vi "EtherNet CIP Write_core.vi"(0 "Connection Cluster":T3={"TCP Connection"=refnum, "Session"=[], "EtherNet/IP Device Address"="172.20.37.243"} {"Session" format="0x%02x"}, 1 "Tag":string, 2 "SINT Array":u8[](array[numeric]), 3 "INT Array":u16[](array[numeric]), 4 "DINT Array":u32[](array[numeric]), 5 "error in":errorcluster, 6 "BOOL Array":bool[](array[boolean]), 7 "REAL Array":sgl[](array[numeric]), 8 "BOOL":bool, 9 "CONTROL/TIMER/COUNTER":T1, 10 "Datatype":T2(ring)) -> (14 "Connection Cluster Out":T3, 19 "error out":errorcluster)   [LabVIEW 2012]
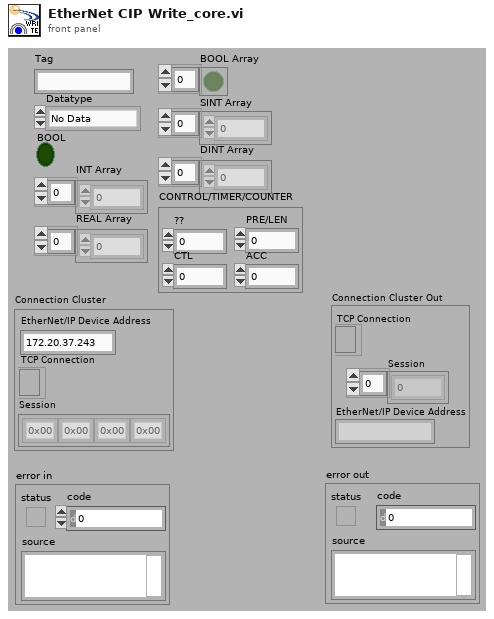
[diagram p1: front panel]
types:
  T1 = cluster{"??":u16, "CTL":u32, "PRE/LEN":u32, "ACC":u32}
  T2 = enum16{"No Data", "BOOL", "BIT Array", "SINT", "INT", "DINT", "REAL", "TIMER/CONTROL/COUNTER"}
  T3 = cluster{"TCP Connection":refnum<k5>, "Session":u8[], "EtherNet/IP Device Address":string}
  T4 = enum16{"Standard", "Buffered", "CRLF", "Immediate"}
  T5 = enum16{"Success", "Unknown Error", "Bad Symbolic Representation", "Item Not Found", "Partial Read", "Error Processing Attribute", "Incorrect/Insufficient Param", "Insufficient Attribute", "Bad Symbolic Length", "Out Of Bound", "Type Mismatch", "Offset Out Of Bound"}
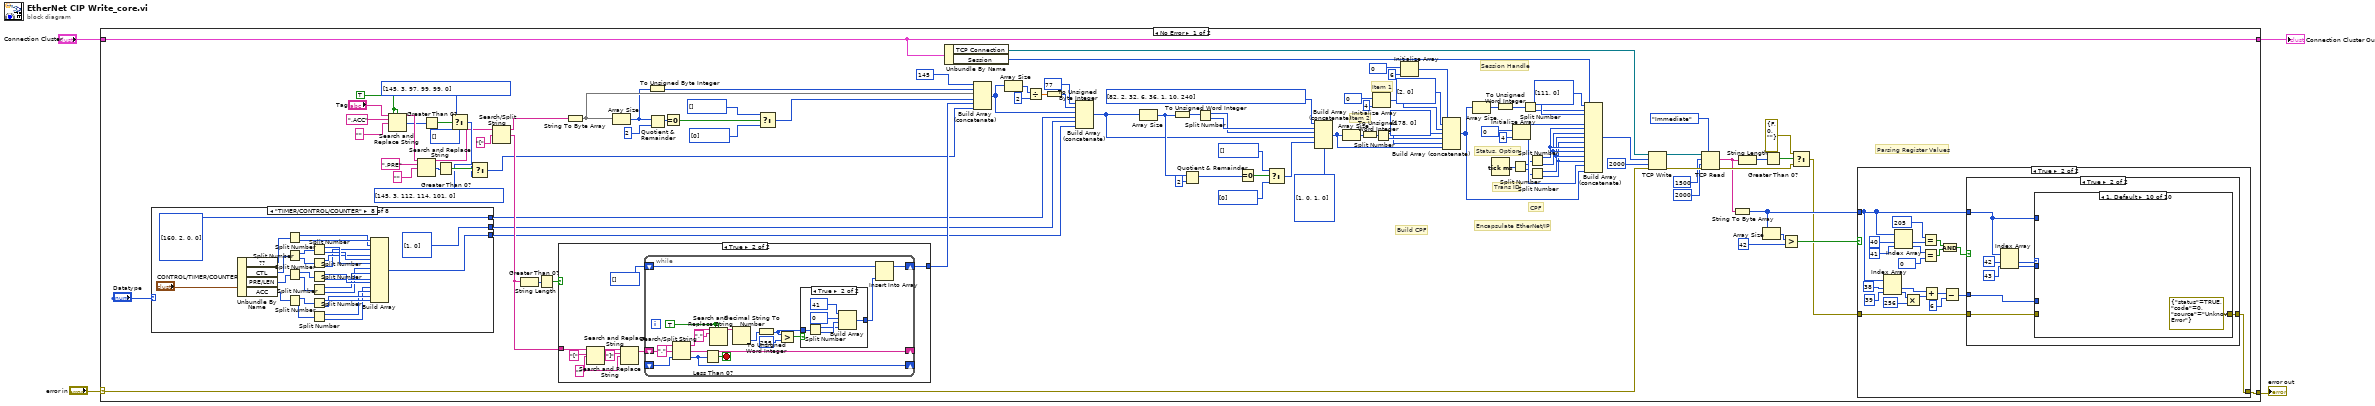
[diagram p0: block diagram]
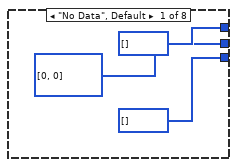
[diagram p2: hidden frame]
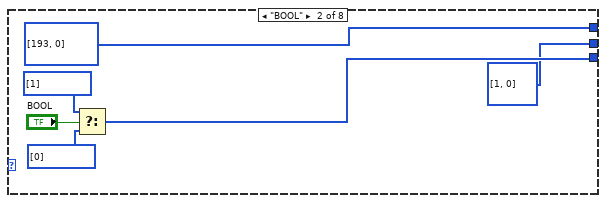
[diagram p3: hidden frame]
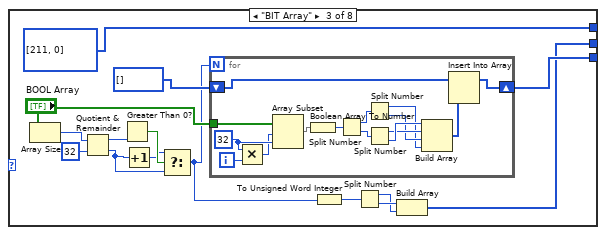
[diagram p4: hidden frame]
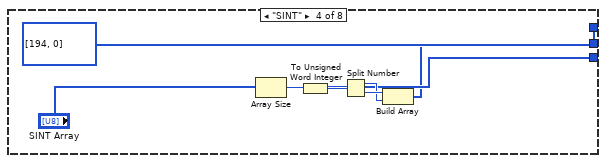
[diagram p5: hidden frame]
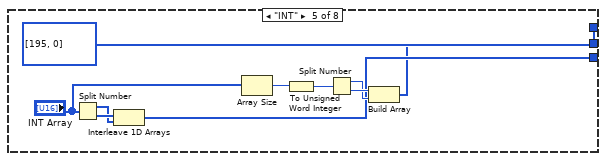
[diagram p6: hidden frame]
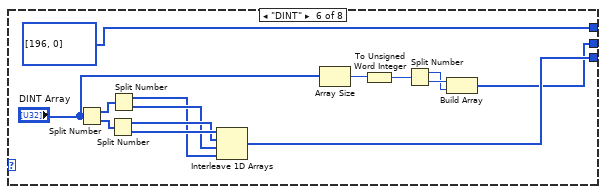
[diagram p7: hidden frame]
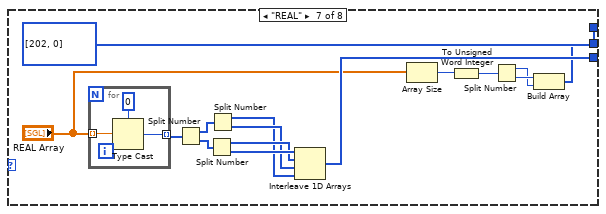
[diagram p8: hidden frame]
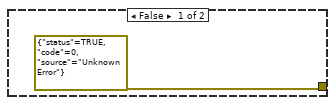
[diagram p9: hidden frame]
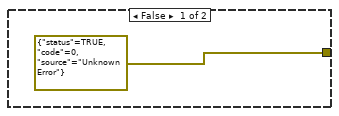
[diagram p10: hidden frame]
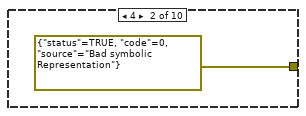
[diagram p12: hidden frame]
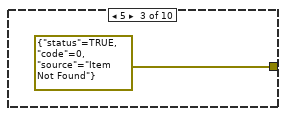
[diagram p13: hidden frame]
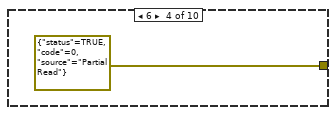
[diagram p14: hidden frame]
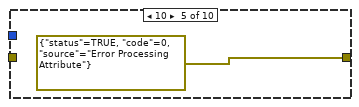
[diagram p15: hidden frame]
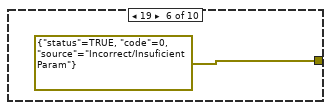
[diagram p16: hidden frame]
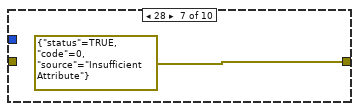
[diagram p17: hidden frame]
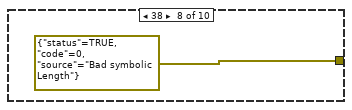
[diagram p18: hidden frame]
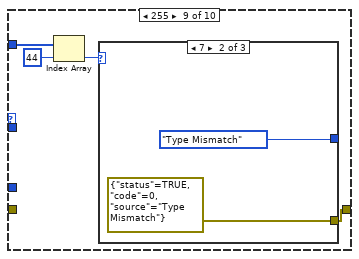
[diagram p19: hidden frame]
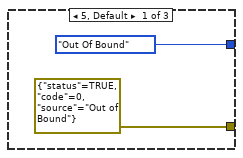
[diagram p20: hidden frame]
diagram:
  n1 = case shown="No Error" "error in" {
    selector: "error in" -> [w6 w315]
    tunnel: "Connection Cluster" -> [w5 w314]
    tunnel: [w8 w315] -> w4
    tunnel: [w5 w314] -> w1
    frame No Error {
      w61 = TRUE ("replace all? (F)")
      # "Parsing Register Values"
      # "Build CPF"
      # "Trans ID"
      # "CPF"
      # "Status, Option"
      # "Session Handle"
      # "Item 2"
      # "Item 1"
      # "Encapsulate EtherNet/IP"
      n2 = case shown="\"TIMER/CONTROL/COUNTER\"" "Datatype" {
        tunnel: [u8[] [] ("SINT Array") w119 w127 "SINT Array" w160 w174 w184 w200] -> w13
        tunnel: [u8[] [] u8[] [193, 0] u8[] [211, 0] u8[] [194, 0] u8[] [195, 0] u8[] [196, 0] u8[] [202, 0] u8[] [160, 2, 0, 0]] -> w14
        tunnel: [u8[] [0, 0] u8[] [1, 0] w123 w151 w159 w173 w183 u8[] [1, 0]] -> w12
        frame "No Data", Default {
        }
        frame "BOOL" {
          n3 = Select(t=u8[] [1], s="BOOL", f=u8[] [0]) -> (s? t:f=w119:u8[])
        }
        frame "BIT Array" {
          n4 = Array Size(array="BOOL Array") -> (size(s)=w122:i32)
          n5 = Quotient & Remainder(x=w122, y=32) -> (x-y*floor(x/y)=w133:i32, floor(x/y)=w131:i32)
          n6 = Greater Than 0?(x=w133) -> (x > 0?=w132:bool)
          n7 = Increment(x=w131) -> (x+1=w130:i32)
          n8 = Select(t=w130, s=w132, f=w131) -> (s? t:f=w121:i32)
          n9 = for {
            N: w121 -> [_]
            tunnel: "BOOL Array" -> [w150]
            shift-right: [w136] -> w127
            shift-left: u8[] [] -> [w138]
            i -> [w149]
            w148 = 32 ("length")
            n10 = Multiply(x=w148, y=w149) -> (x*y=w147:i32)
            n11 = Array Subset(array=w150, index=w147, length=w148) -> (w146:bool[])
            n12 = Boolean Array To Number(Boolean array=w146) -> (number=w145:u32)
            n13 = Split Number(x=w145) -> (hi(x)=w144:u16, lo(x)=w143:u16)
            n14 = Split Number(x=w144) -> (hi(x)=w139:u8, lo(x)=w140:u8)
            n15 = Split Number(x=w143) -> (hi(x)=w141:u8, lo(x)=w142:u8)
            n16 = Build Array(w142, w141, w140, w139) -> (w137:u8[])
            n17 = Insert Into Array(array=w138, new element=w137) -> (w136:u8[])  [unwired: 1 in]
          }
          n18 = To Unsigned Word Integer(number=w121) -> (unsigned 16bit integer=w126:u16)
          n19 = Split Number(x=w126) -> (hi(x)=w124:u8, lo(x)=w125:u8)
          n20 = Build Array(w125, w124) -> (w123:u8[])
        }
        frame "SINT" {
          n21 = Array Size(array="SINT Array") -> (size(s)=w156:i32)
          n22 = To Unsigned Word Integer(number=w156) -> (unsigned 16bit integer=w155:u16)
          n23 = Split Number(x=w155) -> (hi(x)=w153:u8, lo(x)=w154:u8)
          n24 = Build Array(w154, w153) -> (w151:u8[])
        }
        frame "INT" {
          n25 = Split Number(x="INT Array") -> (hi(x)=w165:u8[], lo(x)=w166:u8[])
          n26 = Interleave 1D Arrays(w166, w165) -> (w160:u8[])
          n27 = Array Size(array="INT Array") -> (size(s)=w164:i32)
          n28 = To Unsigned Word Integer(number=w164) -> (unsigned 16bit integer=w163:u16)
          n29 = Split Number(x=w163) -> (hi(x)=w161:u8, lo(x)=w162:u8)
          n30 = Build Array(w162, w161) -> (w159:u8[])
        }
        frame "DINT" {
          n31 = Split Number(x="DINT Array") -> (hi(x)=w180:u16[], lo(x)=w181:u16[])
          n32 = Split Number(x=w181) -> (hi(x)=w170:u8[], lo(x)=w171:u8[])
          n33 = Split Number(x=w180) -> (hi(x)=w168:u8[], lo(x)=w169:u8[])
          n34 = Interleave 1D Arrays(w171, w170, w169, w168) -> (w174:u8[])
          n35 = Array Size(array="DINT Array") -> (size(s)=w178:i32)
          n36 = To Unsigned Word Integer(number=w178) -> (unsigned 16bit integer=w177:u16)
          n37 = Split Number(x=w177) -> (hi(x)=w175:u8, lo(x)=w176:u8)
          n38 = Build Array(w176, w175) -> (w173:u8[])
        }
        frame "REAL" {
          n39 = for {
            tunnel: "REAL Array" -> [w198] mode=indexing
            tunnel: [w197] -> w190 mode=indexing
            n40 = Type Cast(type=u32 0, x=w198) -> (*(type *) &x=w197:u32)
          }
          n41 = Split Number(x=w190) -> (hi(x)=w195:u16[], lo(x)=w196:u16[])
          n42 = Split Number(x=w196) -> (hi(x)=w193:u8[], lo(x)=w194:u8[])
          n43 = Split Number(x=w195) -> (hi(x)=w191:u8[], lo(x)=w192:u8[])
          n44 = Interleave 1D Arrays(w194, w193, w192, w191) -> (w184:u8[])
          n45 = Array Size(array="REAL Array") -> (size(s)=w188:i32)
          n46 = To Unsigned Word Integer(number=w188) -> (unsigned 16bit integer=w187:u16)
          n47 = Split Number(x=w187) -> (hi(x)=w185:u8, lo(x)=w186:u8)
          n48 = Build Array(w186, w185) -> (w183:u8[])
        }
        frame "TIMER/CONTROL/COUNTER" {
          n49 = Unbundle By Name("CONTROL/TIMER/COUNTER") -> ("??"=w225:u16, "CTL"=w224:u32, "PRE/LEN"=w223:u32, "ACC"=w222:u32)
          n50 = Split Number(x=w225) -> (hi(x)=w214:u8, lo(x)=w215:u8)
          n51 = Split Number(x=w224) -> (hi(x)=w221:u16, lo(x)=w220:u16)
          n52 = Split Number(x=w223) -> (hi(x)=w219:u16, lo(x)=w218:u16)
          n53 = Split Number(x=w222) -> (hi(x)=w217:u16, lo(x)=w216:u16)
          n54 = Split Number(x=w221) -> (hi(x)=w213:u8, lo(x)=w212:u8)
          n55 = Split Number(x=w220) -> (hi(x)=w211:u8, lo(x)=w210:u8)
          n56 = Split Number(x=w219) -> (hi(x)=w209:u8, lo(x)=w208:u8)
          n57 = Split Number(x=w218) -> (hi(x)=w207:u8, lo(x)=w206:u8)
          n58 = Split Number(x=w217) -> (hi(x)=w205:u8, lo(x)=w204:u8)
          n59 = Split Number(x=w216) -> (hi(x)=w203:u8, lo(x)=w202:u8)
          n60 = Build Array(w215, w214, w210, w211, w212, w213, w206, w207, w208, w209, w202, w203, w204, w205) -> (w200:u8[])
        }
      }
      n61 = Search and Replace String(replace all?=w61, case sensitive?=w61, input string="Tag", search string=".ACC", replace string="" ("replace string (\"\")")) -> (result string=w58:string, number of replacements=w57:i32)  [unwired: 3 in, 2 out]
      n62 = Search and Replace String(input string=w58, search string=".PRE", replace string="" ("replace string (\"\")")) -> (result string=w48:string, number of replacements=w56:i32)  [unwired: 5 in, 2 out]
      n63 = Greater Than 0?(x=w57) -> (x > 0?=w55:bool)
      n64 = Greater Than 0?(x=w56) -> (x > 0?=w54:bool)
      n65 = Select(t=u8[] [145, 3, 97, 99, 99, 0], s=w55, f=u8[] []) -> (s? t:f=w51:u8[])
      n66 = Select(t=u8[] [145, 3, 112, 114, 101, 0], s=w54, f=w51) -> (s? t:f=w26:u8[])
      n67 = Search/Split String(string=w48, search string/char (-)="[") -> (substring before match=w47:string, match + rest of string=w28:string)  [unwired: 1 in, 1 out]
      n68 = String Length(string=w28) -> (length=w30:i32)
      n69 = Greater Than 0?(x=w30) -> (x > 0?=w29:bool)
      n70 = case shown="True" w29 {
        tunnel: w28 -> [_ w280]
        tunnel: [u8[] [] w279] -> w27
        frame False {
        }
        frame True {
          w283 = "" ("replace string (\"\")")
          n71 = Search and Replace String(input string=w280, search string="[", replace string=w283) -> (result string=w285:string)  [unwired: 5 in, 3 out]
          n72 = Search and Replace String(input string=w285, search string="]", replace string=w283) -> (result string=w282:string)  [unwired: 5 in, 3 out]
          n73 = while {
            shift-right: [w296] -> _
            shift-left: _ -> [w303]
            shift-right: [w301] -> _
            shift-left: w282 -> [w302]
            shift-right: [w288] -> w279
            shift-left: u8[] [] -> [w290]
            stop <- w297 stop-if-true
            w295 = TRUE ("replace all? (F)")
            n74 = Search/Split String(string=w302, search string/char (-)=",", offset (0)=w303) -> (substring before match=w299:string, match + rest of string=w301:string, offset of match=w296:i32)
            n75 = Less Than 0?(x=w296) -> (x < 0?=w297:bool)
            n76 = Search and Replace String(replace all?=w295, case sensitive?=w295, input string=w299, search string=",") -> (result string=w294:string)  [unwired: 4 in, 3 out]
            n77 = Decimal String To Number(string=w294) -> (number=w291:i32)  [unwired: 2 in, 1 out]
            n78 = To Unsigned Word Integer(number=w291) -> (unsigned 16bit integer=w287:u16)
            n79 = Greater?(x=w287, y=u16 255) -> (0:w292:bool)
            n80 = case shown="True" w292 {
              tunnel: w287 -> [w307 w313]
              tunnel: [w304 w308] -> w289
              frame False {
                n81 = To Unsigned Byte Integer(number=w307) -> (unsigned 8bit integer=w306:u8)
                n82 = Build Array(u8 40 ("Status"), w306) -> (w304:u8[])
              }
              frame True {
                n83 = Split Number(x=w313) -> (hi(x)=w311:u8, lo(x)=w312:u8)
                n84 = Build Array(u8 41 ("Status"), u8 0 ("Status"), w312, w311) -> (w308:u8[])
              }
            }
            n85 = Insert Into Array(array=w290, new element=w289) -> (w288:u8[])  [unwired: 1 in]
          }
        }
      }
      n86 = String To Byte Array(string=w47) -> (unsigned byte array=w45:u8[])
      n87 = Array Size(array=w45) -> (size(s)=w32:i32)
      n88 = To Unsigned Byte Integer(number=w32) -> (unsigned 8bit integer=w44:u8)
      n89 = Quotient & Remainder(x=w32, y=2) -> (x-y*floor(x/y)=w34:i32)  [unwired: 1 out]
      n90 = Equal To 0?(x=w34) -> (x = 0?=w37:bool)
      n91 = Select(t=u8[] [], s=w37, f=u8[] [0]) -> (s? t:f=w31:u8[])
      n92 = Unbundle By Name(w5) -> ("TCP Connection"=w108:refnum<k5>, "Session"=w94:u8[])
      n93 = Build Array (concatenate)(u8 145 ("Status"), w44, w45, w31, w27, w26) -> (w23:u8[])
      n94 = Array Size(array=w23) -> (size(s)=w11:i32)
      n95 = Divide(x=w11, y=u8 2) -> (x/y=w9:dbl)
      n96 = To Unsigned Byte Integer(number=w9) -> (unsigned 8bit integer=w24:u8)
      n97 = Build Array (concatenate)(u8 77 ("Status"), w24, w23, w14, w12, w13) -> (w22:u8[])
      n98 = Array Size(array=w22) -> (size(s)=w38:i32)
      n99 = To Unsigned Word Integer(number=w38) -> (unsigned 16bit integer=w106:u16)
      n100 = Quotient & Remainder(x=w38, y=2) -> (x-y*floor(x/y)=w65:i32)  [unwired: 1 out]
      n101 = Split Number(x=w106) -> (hi(x)=w104:u8, lo(x)=w105:u8)
      n102 = Equal To 0?(x=w65) -> (x = 0?=w40:bool)
      n103 = Select(t=u8[] [], s=w40, f=u8[] [0]) -> (s? t:f=w39:u8[])
      n104 = Build Array (concatenate)(u8[] [82, 2, 32, 6, 36, 1, 10, 240], w105, w104, w22, w39, u8[] [1, 0, 1, 0]) -> (w67:u8[])
      n105 = Array Size(array=w67) -> (size(s)=w71:i32)
      n106 = To Unsigned Word Integer(number=w71) -> (unsigned 16bit integer=w72:u16)
      n107 = Initialize Array(u8 0 ("Status"), 4 ("dimension size")) -> (w69:u8[])
      n108 = Split Number(x=w72) -> (hi(x)=w68:u8, lo(x)=w70:u8)
      n109 = Initialize Array(u8 0 ("Status"), 6 ("dimension size")) -> (w75:u8[])
      n110 = Build Array (concatenate)(w75, u8[] [2, 0], w69, u8[] [178, 0], w70, w68, w67) -> (w21:u8[])
      n111 = Array Size(array=w21) -> (size(s)=w100:i32)
      n112 = Tick Count (ms)() -> (millisecond timer value=w93:u32)
      n113 = To Unsigned Word Integer(number=w100) -> (unsigned 16bit integer=w101:u16)
      n114 = Split Number(x=w93) -> (hi(x)=w92:u16, lo(x)=w91:u16)
      n115 = Initialize Array(u8 0 ("Status"), 4 ("dimension size")) -> (w95:u8[])
      n116 = Split Number(x=w101) -> (hi(x)=w99:u8, lo(x)=w98:u8)
      n117 = Split Number(x=w92) -> (hi(x)=w90:u8, lo(x)=w89:u8)
      n118 = Split Number(x=w91) -> (hi(x)=w88:u8, lo(x)=w87:u8)
      n119 = Build Array (concatenate)(u8[] [111, 0], w98, w99, w94, w95, w90, w89, w88, w87, w90, w89, w88, w87, w95, w21) -> (w86:u8[])
      n120 = TCP Write(connection ID=w108, data in=w86, error in (no error)=w6, 9:2000 ("timeout ms (25000)")) -> (connection ID out=w110:refnum<k5>, error out=w111:errorcluster)  [unwired: 1 out]
      n121 = TCP Read(connection ID=w110, bytes to read=1500, error in (no error)=w111, 7:T4."Immediate" ("mode (standard)"), 9:2000 ("timeout ms (25000)")) -> (data out=w80:string, error out=w81:errorcluster)  [unwired: 1 out]
      n122 = String To Byte Array(string=w80) -> (unsigned byte array=w16:u8[])
      n123 = String Length(string=w80) -> (length=w84:i32)
      n124 = Array Size(array=w16) -> (size(s)=w19:i32)
      n125 = Greater Than 0?(x=w84) -> (x > 0?=w83:bool)
      n126 = Greater?(x=w19, y=42) -> (0:w17:bool)
      n127 = Select(t=errorcluster {"status"=FALSE, "code"=0, "source"=""} ("error IO"), s=w83, f=w81) -> (s? t:f=w7:errorcluster)
      n128 = case shown="True" w17 {
        tunnel: w16 -> [_ w240]
        tunnel: [errorcluster {"status"=TRUE, "code"=0, "source"="Unknown Error"} ("error out") w230] -> w8
        tunnel: w7 -> [_ w229]
        frame False {
        }
        frame True {
          n129 = Index Array(array=w240, index #1=38 ("index"), index #2=39 ("index")) -> (element #1=w234:u8, element #2=w237:u8)
          n130 = Index Array(array=w240, index #1=40 ("index"), index #2=41 ("index")) -> (element #1=w246:u8, element #2=w247:u8)
          n131 = Multiply(x=w237, y=u16 256) -> (x*y=w235:u16)
          n132 = Equal?(x=u8 205 ("Status"), y=w246) -> (x = y?=w242:bool)
          n133 = Equal?(x=w247, y=u8 0 ("Status")) -> (x = y?=w243:bool)
          n134 = Add(x=w234, y=w235) -> (x+y=w233:u16)
          n135 = And(x=w242, y=w243) -> (x .and. y?=w241:bool)
          n136 = Subtract(x=w233, y=u16 6) -> (x-y=w231:u16)
          n137 = case shown="True" w241 {
            tunnel: w240 -> [_ w255]
            tunnel: w231 -> [_ w254]
            tunnel: [errorcluster {"status"=TRUE, "code"=0, "source"="Unknown Error"} ("error out") w252] -> w230
            tunnel: w229 -> [_ w251]
            frame False {
            }
            frame True {
              n138 = Index Array(array=w255, index #1=42 ("index"), index #2=43 ("index")) -> (element #1=w256:u8, element #2=w253:u8)
              n139 = case shown="1, Default" w256 {
                tunnel: w253 -> [_ _ _ _ _ _ _ _ _ _]
                tunnel: w255 -> [_ _ _ _ _ _ _ _ w270 _]
                tunnel: w254 -> [_ _ _ _ _ _ _ _ _ _]
                tunnel: [w259 errorcluster {"status"=TRUE, "code"=0, "source"="Bad symbolic Representation"} ("error out") errorcluster {"status"=TRUE, "code"=0, "source"="Item Not Found"} ("error out") errorcluster {"status"=TRUE, "code"=0, "source"="Partial Read"} ("error out") errorcluster {"status"=TRUE, "code"=0, "source"="Error Processing Attribute"} ("error out") errorcluster {"status"=TRUE, "code"=0, "source"="Incorrect/Insuficient Param"} ("error out") errorcluster {"status"=TRUE, "code"=0, "source"="Insufficient Attribute"} ("error out") errorcluster {"status"=TRUE, "code"=0, "source"="Bad symbolic Length"} ("error out") w267 errorcluster {"status"=TRUE, "code"=0, "source"="Unknown Error"} ("error out")] -> w252
                tunnel: w251 -> [w259 _ _ _ _ _ _ _ _ _]
                frame 0 {
                }
                frame 4 {
                }
                frame 5 {
                }
                frame 6 {
                }
                frame 10 {
                }
                frame 19 {
                }
                frame 28 {
                }
                frame 38 {
                }
                frame 255 {
                  n140 = Index Array(array=w270, index=44) -> (element=w268:u8)
                  n141 = case shown="7" w268 {
                    tunnel: [T5."Out Of Bound" ("Status") T5."Type Mismatch" ("Status") T5."Offset Out Of Bound" ("Status")] -> _
                    tunnel: [errorcluster {"status"=TRUE, "code"=0, "source"="Out of Bound"} ("error out") errorcluster {"status"=TRUE, "code"=0, "source"="Type Mismatch"} ("error out") errorcluster {"status"=TRUE, "code"=0, "source"="Offset Out Of Bound"} ("error out")] -> w267
                    frame 5, Default {
                    }
                    frame 7 {
                    }
                    frame 4 {
                    }
                  }
                }
                frame 1, Default {
                }
              }
            }
          }
        }
      }
    }
    frame Error {
      (unwired) u16[] []
    }
  }
  "error out" <- w4
  "Connection Cluster Out" <- w1
